vi "Update GU Arrange List.vi"(8 "error in":errorcluster, 10 "Curr Cal Cfg":T1, 11 "Ctrl Ref":T2) -> (0 "error out":errorcluster)   [LabVIEW 2020, in "GUCalibration2.lvlib"]
uses:
  GUCalibration2.lvlib
  Controls/GU Arrange UI Ref.ctl
  Controls/Config Data Type.ctl
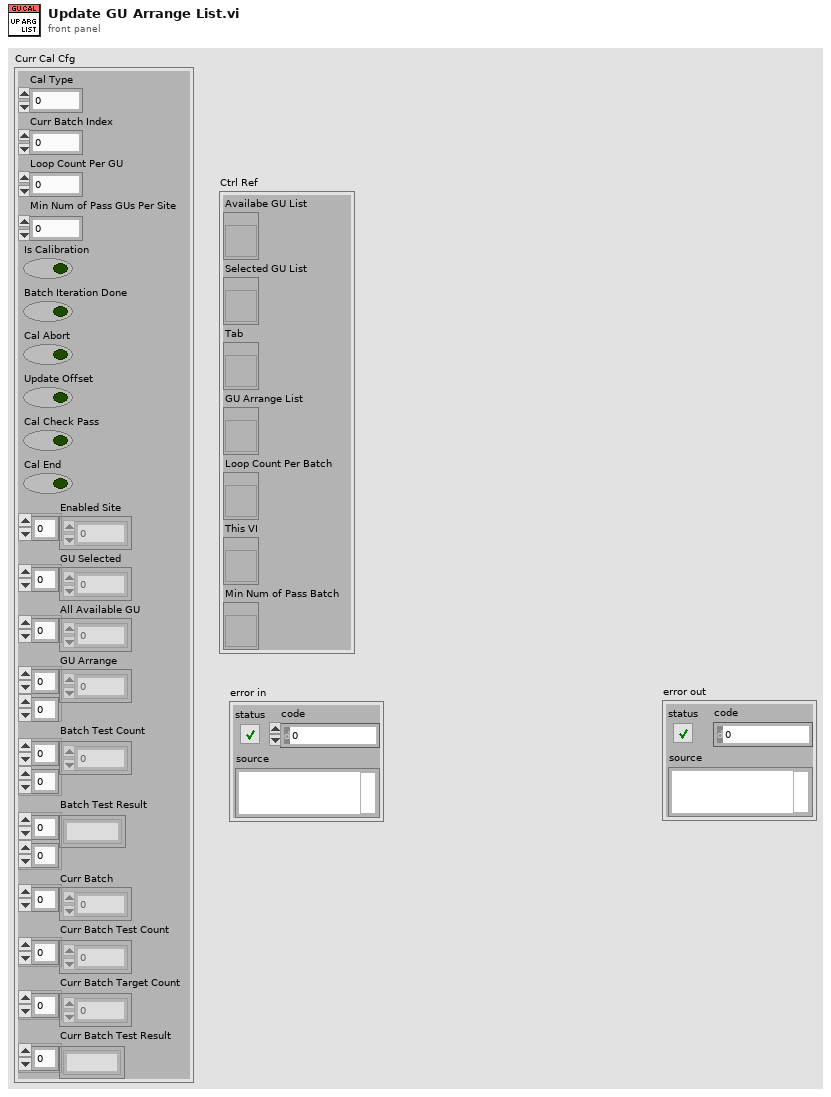
[diagram p1: front panel]
types:
  T1 = typedef "GUCalibration2.lvlib/Config Data Type.ctl" = cluster{"Cal Type":i32, "Curr Batch Index":i32, "Loop Count Per GU":i32, "Min Num of Pass GUs Per Site":i32, "Is Calibration":bool, "Batch Iteration Done":bool, "Cal Abort":bool, "Update Offset":bool, "Cal Check Pass":bool, "Cal End":bool, "Enabled Site":i32[], "GU Selected":i32[], "All Available GU":i32[], "GU Arrange":i32[][], "Batch Test Count":i32[][], "Batch Test Result":string[][], "Curr Batch":i32[], "Curr Batch Test Count":i32[], "Curr Batch Target Count":i32[], "Curr Batch Test Result":string[]}
  T2 = typedef "GUCalibration2.lvlib/GU Arrange UI Ref.ctl" = cluster{"Availabe GU List":refnum<vi>, "Selected GU List":refnum<vi>, "Tab":refnum<vi>, "GU Arrange List":refnum<vi>, "Loop Count Per Batch":refnum<vi>, "This VI":refnum<vi>, "Min Num of Pass Batch":refnum<vi>}
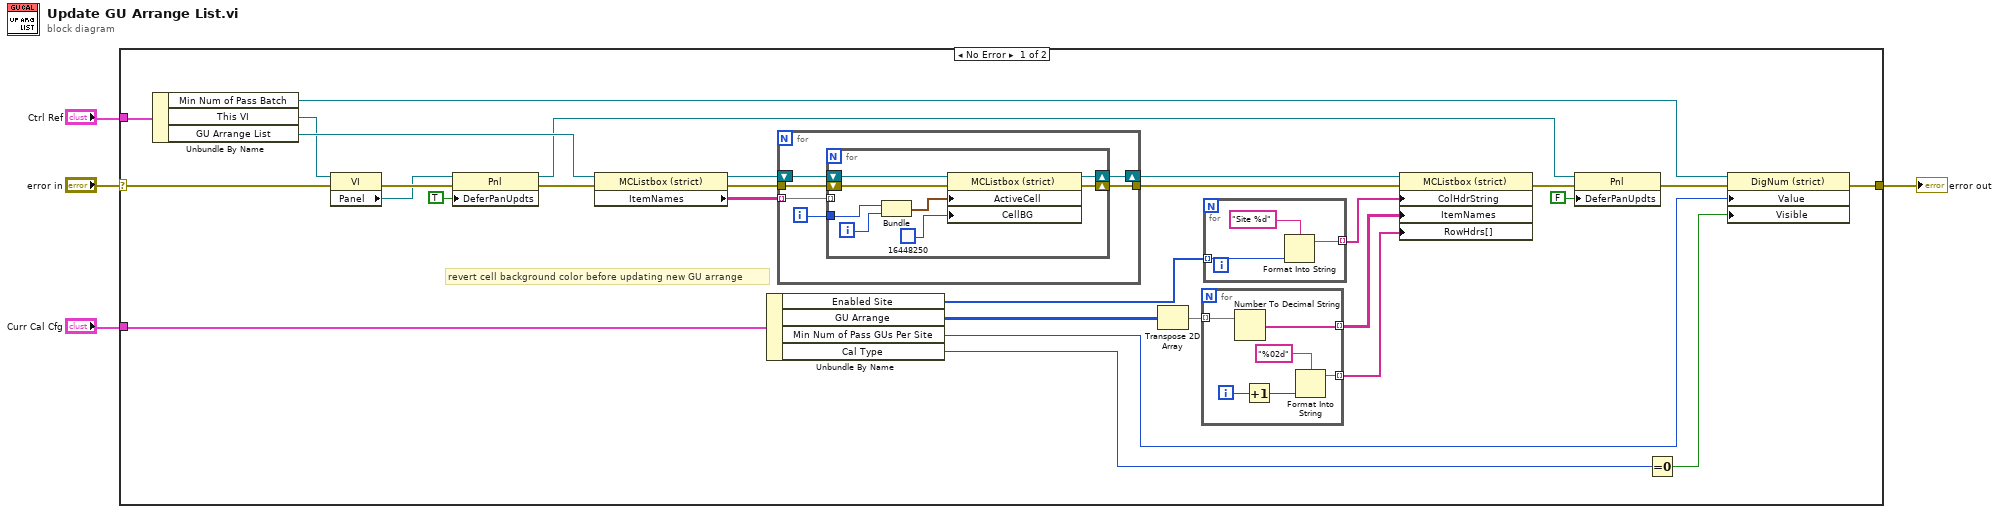
[diagram p0: block diagram]
diagram:
  n1 = case shown="No Error" "error in" {
    selector: "error in" -> [w20 w57]
    tunnel: "Ctrl Ref" -> [w33 _]
    tunnel: "Curr Cal Cfg" -> [w32 _]
    tunnel: [w8 w57] -> w2
    frame No Error {
      # "revert cell background color before updating new GU arrange"
      n2 = Unbundle By Name(w33) -> ("Min Num of Pass Batch"=w11:refnum<vi>, "This VI"=w17:refnum<vi>, "GU Arrange List"=w21:refnum<vi>)
      n3 = property class="VI"(reference=w17, error in=w20) -> (error out=w28:errorcluster, "Panel"=w27:refnum<vi>)  [unwired: 1 out]
      n4 = property class="Pnl"(reference=w27, error in=w28, "DeferPanUpdts"=TRUE ("Defer Panel Updates")) -> (reference out=w13:refnum<vi>, error out=w19:errorcluster)
      n5 = property class="MCListbox (strict)"(reference=w21, error in=w19) -> (reference out=w16:refnum<vi>, error out=w15:errorcluster, "ItemNames"=w18:string[][])
      n6 = Unbundle By Name(w32) -> ("Enabled Site"=w24:i32[], "GU Arrange"=w31:i32[][], "Min Num of Pass GUs Per Site"=w9:i32, "Cal Type"=w7:i32)
      n7 = for {
        tunnel: w18 -> [w35] mode=indexing
        tunnel: w15 -> [w38]
        tunnel: [w37] -> w14
        shift-right: [w34] -> w12
        shift-left: w16 -> [w39]
        i -> [w36]
        n8 = for {
          shift-right: [w45] -> w37
          shift-left: w38 -> [w46]
          tunnel: w36 -> [w44]
          tunnel: w35 -> [_] mode=indexing
          shift-right: [w40] -> w34
          shift-left: w39 -> [w47]
          i -> [w43]
          n9 = Bundle(w44, w43) -> (w42:cluster{i32, i32})  [unwired: 1 in]
          n10 = property class="MCListbox (strict)"(reference=w47, error in=w46, "ActiveCell"=w42, "CellBG"=u32 16448250) -> (reference out=w40:refnum<vi>, error out=w45:errorcluster)
        }
      }
      n11 = Transpose 2D Array(2D array=w31) -> (transposed array=w22:i32[][])
      n12 = for {
        tunnel: w22 -> [w56] mode=indexing
        tunnel: [w55] -> w29 mode=indexing
        tunnel: [w53] -> w30 mode=indexing
        i -> [w54]
        n13 = Number To Decimal String(number=w56) -> (decimal integer string=w55:string[])  [unwired: 1 in]
        n14 = Increment(x=w54) -> (x+1=w51:i32)
        n15 = Format Into String(format string="%02d", w51) -> (resulting string=w53:string)  [unwired: 2 in, 1 out]
      }
      n16 = for {
        tunnel: w24 -> [w49] mode=indexing
        tunnel: [w48] -> w23 mode=indexing
        n17 = Format Into String(format string="Site %d", w49) -> (resulting string=w48:string)  [unwired: 2 in, 1 out]
      }
      n18 = property class="MCListbox (strict)"(reference=w12, error in=w14, "ColHdrString"=w23, "ItemNames"=w29, "RowHdrs[]"=w30) -> (error out=w5:errorcluster)  [unwired: 1 out]
      n19 = property class="Pnl"(reference=w13, error in=w5, "DeferPanUpdts"=FALSE ("Defer Panel Updates")) -> (error out=w10:errorcluster)  [unwired: 1 out]
      n20 = Equal To 0?(x=w7) -> (x = 0?=w6:bool)
      n21 = property class="DigNum (strict)"(reference=w11, error in=w10, "Value"=w9, "Visible"=w6) -> (error out=w8:errorcluster)  [unwired: 1 out]
    }
    frame Error {
    }
  }
  "error out" <- w2
